vi "Read ListBox.vi"(8 "error in (no error)":errorcluster, 11 "Popup in":refnum<class "Popup.lvclass">) -> (0 "error out":errorcluster, 2 "ListBox":refnum<vi>, 3 "Popup out":refnum<class "Popup.lvclass">)   [LabVIEW 2017, in "Popup.lvclass"]
uses:
  Popup.lvclass
  Popup.lvclass/Popup.ctl
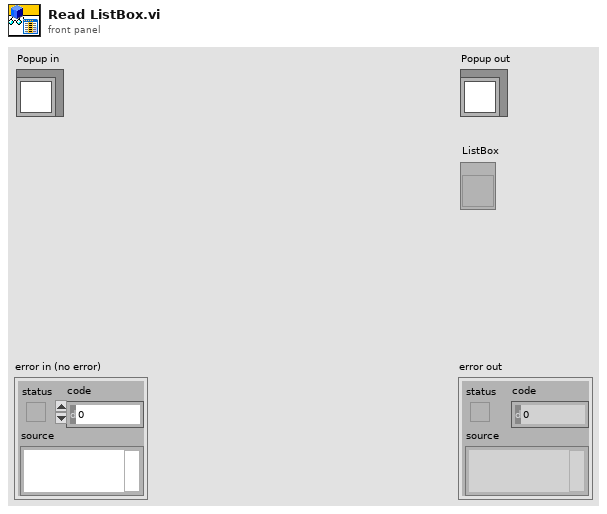
[diagram p1: front panel]
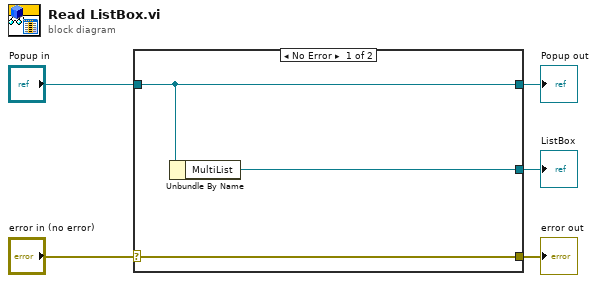
[diagram p0: block diagram]
diagram:
  n1 = case shown="No Error" "error in (no error)" {
    selector: "error in (no error)" -> [w8 w9]
    tunnel: [w8 w9] -> w4
    tunnel: [w7 w10] -> w2
    tunnel: "Popup in" -> [w7 w10]
    tunnel: [w6 _] -> w1
    frame No Error {
      n2 = Unbundle By Name(w7) -> ("MultiList"=w6:refnum<vi>)
    }
    frame Error {
    }
  }
  "error out" <- w4
  "Popup out" <- w2
  "ListBox" <- w1
